vi "ArduinoLeonardoReadDI.vi"(8 "error in (no error)":errorcluster, 10 "default":refnum<visa-resource-name>, 11 "VISA resource name":refnum<visa-resource-name>) -> (0 "error out":errorcluster, 2 "Buttons":bool[](array[boolean]), 3 "VISA resource name out":refnum<visa-resource-name>)   [LabVIEW 2014]
doc: "read Buttons status from Arduino:\n0-4: preset heights\n5: container offset\n6-8: offsets(step, platform, ground)\n9: drop\n10-11: fork opening (close/Wide)\n12: reset"
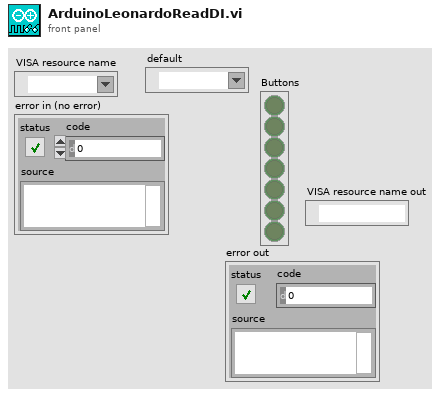
[diagram p1: front panel]
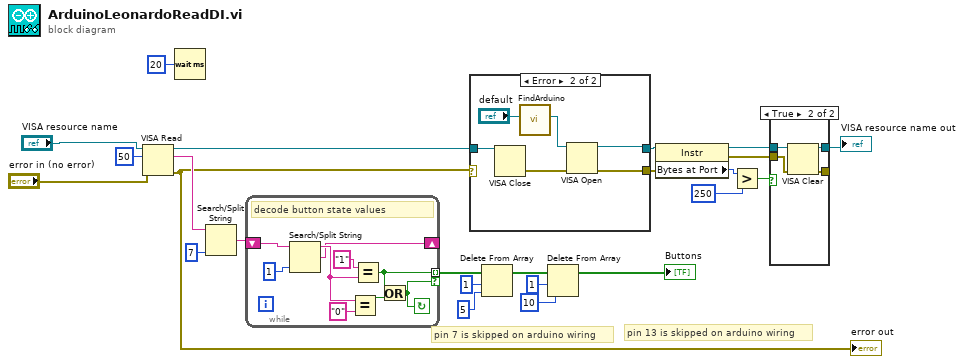
[diagram p0: block diagram]
diagram:
  # "pin 13 is skipped on arduino wiring"
  # "pin 7 is skipped on arduino wiring"
  n1 = VISA Read(VISA resource name="VISA resource name", byte count=u32 50, error in (no error)="error in (no error)") -> (VISA resource name out=w10:refnum<visa-resource-name>, read buffer=w22:string, error out=w9:errorcluster)  [unwired: 1 out]
  "error out" <- w9
  n2 = Wait (ms)(milliseconds to wait=u32 20) -> ()  [unwired: 1 out]
  n3 = Search/Split String(string=w22, offset (0)=7) -> (match + rest of string=w20:string)  [unwired: 1 in, 2 out]
  n4 = while {
    tunnel: [w28] -> w6 mode=indexing if=w27
    shift-right: [w25] -> _
    shift-left: w20 -> [w33]
    stop <- w27 continue-if-true
    # "decode button state values"
    n5 = Search/Split String(string=w33, offset (0)=1 ("length (rest)")) -> (substring before match=w26:string, match + rest of string=w25:string)  [unwired: 1 in, 1 out]
    n6 = Equal?(x=w26, y="0") -> (x = y?=w29:bool)
    n7 = Equal?(x="1" ("y"), y=w26) -> (x = y?=w28:bool)
    n8 = Or(x=w28, y=w29) -> (x .or. y?=w27:bool)
  }
  n9 = case shown="Error" w9 {
    selector: w9 -> [w34 _]
    tunnel: [w35 w39] -> w18
    tunnel: w10 -> [w35 w40]
    tunnel: [w34 w38] -> w11
    frame No Error {
    }
    frame Error {
      n10 = VISA Close(VISA resource name=w40) -> (error out=w41:errorcluster)  [unwired: 1 in]
      n11 = call "FindArduino.vi"("default"="default") -> ("VISA resource name"=w37:refnum<visa-resource-name>)  [unwired: 10 in]
      n12 = VISA Open(error in (no error)=w41, VISA resource name=w37) -> (VISA resource name=w39:refnum<visa-resource-name>, error out=w38:errorcluster)  [unwired: 3 in]
    }
  }
  n13 = Delete From Array(array=w6, length=1, index=5) -> (array with subset deleted=w7:bool[])  [unwired: 1 out]
  n14 = Delete From Array(array=w7, length=1, index=10) -> (array with subset deleted=→"Buttons":bool[])  [unwired: 1 out]
  n15 = property class="Instr"(reference=w18, error in=w11) -> (reference out=w16:refnum<visa-resource-name>, error out=w12:errorcluster, "Bytes at Port"=w15:u32)
  n16 = Greater?(x=w15, y=u32 250) -> (0:w13:bool)
  n17 = case shown="True" w13 {
    tunnel: [w43 w47] -> w17
    tunnel: w16 -> [w43 w46]
    tunnel: w12 -> [w42 w44]
    tunnel: [w42 w45] -> _
    frame False {
    }
    frame True {
      n18 = VISA Clear(VISA resource name=w46, error in (no error)=w44) -> (VISA resource name out=w47:refnum<visa-resource-name>, error out=w45:errorcluster)
    }
  }
  "VISA resource name out" <- w17
